vi "RichToFlatcif_manager_CreateOrchRequest.vi"(5 "OutputClusterType":T1, 11 "InputCluster":T3) -> (3 "OutputCluster":T1)   [LabVIEW 2021, in "CIF_Manager_client.lvlib"]
uses:
  CIF_Manager_client.lvlib
  cif_manager_CreateOrchRequest.ctl
  cif_manager_OrchestrationLanguage.ctl
  cif_manager_CreateOrchRequest_Flat.ctl
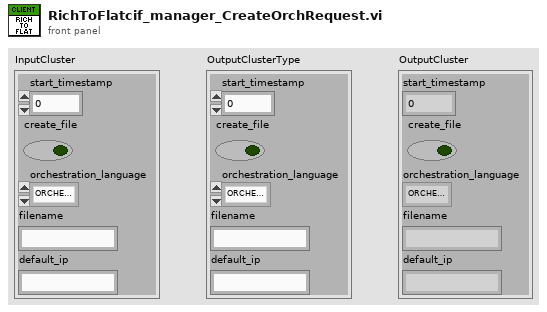
[diagram p1: front panel]
types:
  T1 = typedef "CIF_Manager_client.lvlib/cif_manager_CreateOrchRequest_Flat.ctl" = cluster{"start_timestamp":u64, "create_file":bool, "orchestration_language":T2, "filename":string, "default_ip":string}
  T2 = typedef "CIF_Manager_client.lvlib/cif_manager_OrchestrationLanguage.ctl" = enum32{"ORCHESTRATIONLANGUAGE_UNKNOWN", "ORCHESTRATIONLANGUAGE_PYTHON"}
  T3 = typedef "CIF_Manager_client.lvlib/cif_manager_CreateOrchRequest.ctl" = cluster{"start_timestamp":u64, "create_file":bool, "orchestration_language":T2, "filename":string, "default_ip":string}
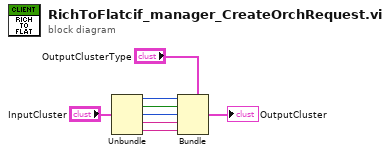
[diagram p0: block diagram]
diagram:
  n1 = Unbundle "Unbundle"("InputCluster") -> ("start_timestamp"=w5:u64, "create_file"=w4:bool, "orchestration_language"=w3:T2, "filename"=w2:string, "default_ip"=w1:string)
  n2 = Bundle "Bundle"(cluster="OutputClusterType", "start_timestamp"=w5, "create_file"=w4, "orchestration_language"=w3, "filename"=w2, "default_ip"=w1) -> (→"OutputCluster":T1)
